vi "usrp tx new.vi"() -> ()   [LabVIEW 2014]
uses:
  <instrlib>/niUSRP/niUSRP Write Tx Data (CDB WDT).vi
  <vilib>/measure/NI_MABase.lvlib
panel:
  in  "gain 2":dbl format="%#_6f"
  in  "active antenna":string
  in  "carrier frequency 2":dbl=100000.0 format="%#_6p"
  in  "IQ rate 2":dbl=100000.0 format="%#_6p"
  in  "stop 2":bool
  in  "frequency 2":dbl=10.0 format="%0.2p"
  in  "signal type 2":T1(ring)
  out "Waveform Graph 2":waveform(dbl)(graph)
  in  "device names 2":refnum<k15>
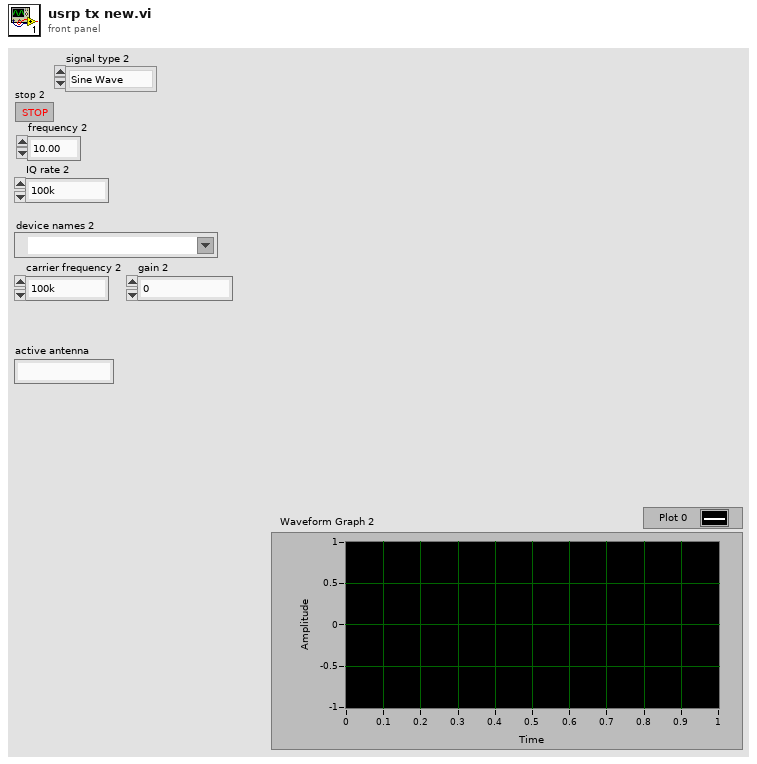
[diagram p1: front panel]
types:
  T1 = enum16{"Sine Wave", "Triangle Wave", "Square Wave", "Sawtooth Wave"}
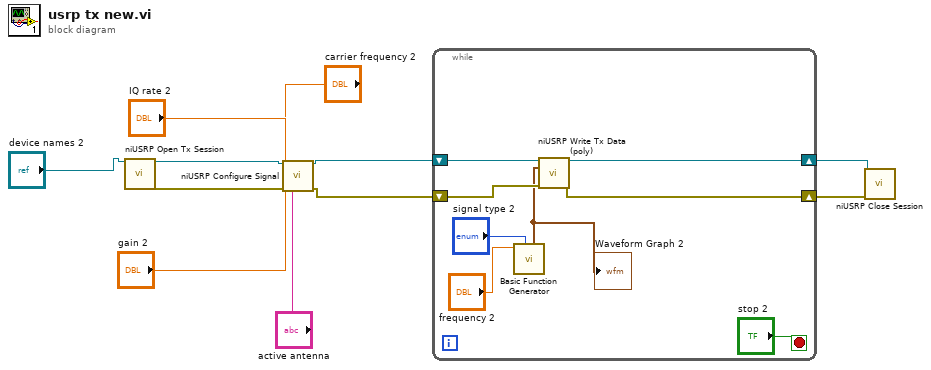
[diagram p0: block diagram]
diagram:
  n1 = call <instrlib>:"niUSRP Open Tx Session.vi"("device names"="device names 2") -> ("session handle out"=w10:refnum<k15>, "error out"=w5:errorcluster)  [unwired: 13 in]
  n2 = call <instrlib>:"niUSRP Configure Signal.vi"("session handle"=w10, "IQ rate"="IQ rate 2", "carrier frequency"="carrier frequency 2", "gain"="gain 2", "error in (no error)"=w5, "active antenna"="active antenna") -> ("session handle out"=w9:refnum<k15>, "error out"=w6:errorcluster)  [unwired: 5 in, 3 out]
  n3 = while {
    shift-right: [w18] -> w8
    shift-left: w9 -> [w19]
    shift-right: [w17] -> w7
    shift-left: w6 -> [w16]
    stop <- "stop 2" stop-if-true
    n4 = call <vilib>:"Basic Function Generator.vi"("signal type"="signal type 2", "frequency"="frequency 2") -> ("signal out"=w12:waveform(dbl))  [unwired: 7 in, 2 out]
    "Waveform Graph 2" <- w12
    n5 = call-poly <instrlib>:"niUSRP Write Tx Data (poly).vi"("session handle"=w19, "data"=w12, "error in (no error)"=w16) -> ("session handle out"=w18:refnum<k15>, "error out"=w17:errorcluster)  [unwired: 11 in]
  }
  n6 = call <instrlib>:"niUSRP Close Session.vi"("session handle"=w8, "error in (no error)"=w7) -> ()  [unwired: 13 in, 1 out]
